vi "medicaoIXV.vi"(0 "Nome da célula":string, 1 "Tipo":string caption="Tipo da célula", 2 "p.d.j":dbl caption="Pontos depois do joelho", 3 "temperatura":dbl caption="Temperatura da célula" format="%#_3g", 4 "nMedições":i16=1 caption="N° medições por ponto" min=1, 5 "Formato":u16(ring) items=[".txt", ".csv"], 6 "nCurvas":i64=1 caption="Nº de curvas" min=1, 7 "p.a.j":dbl caption="Pontos antes do joelho", 8 "Delay(ms)":dbl, 9 "Local":path, 10 "Start":bool, 11 "T.J":dbl caption="Tensão do joelho" step=0.1, 12 "area":dbl caption="Área da célula(cm²)", 13 "Irradiância":dbl caption="Irradiância(W/cm²)", 14 "T.M":dbl caption="Tensão máxima" step=0.1, 15 "print?":bool) -> ()   [LabVIEW 2012]
uses:
  <vilib>/silver_ctls/ArrayMatrixCluster/Real Matrix NI_Silver.ctl
  <vilib>/Utility/file.llb/Write To Spreadsheet File (string).vi
  <vilib>/Utility/file.llb/Write To Spreadsheet File (DBL).vi
  <instrlib>/Agilent 6XXX Series/Agilent 6XXX Series.lvlib
  <vilib>/Analysis/NI_AALBase.lvlib
panel:
  out "Curva atual":dbl
  in  "correcao":bool caption="Correção da curva"
  in  "stopProgram":bool caption="Realizar outra medição"
  out "ON/OFF1":bool caption="ON/OFF"
  out "tensaoFonte":dbl caption="Tensão da fonte (V)"
  out "Temp":dbl caption="Temperatura da célula (°C)" format="%#_3g"
  out "Imp":dbl caption="Imp(A)"
  out "Vmp":dbl caption="Vmp(V)"
  out "Pmp":dbl caption="Pmp(W)"
  out "Icc (A)":dbl
  out "Vca (V)":dbl
  out "IXV":cluster{"Y":dbl[], "Y":dbl[]}[](graph)
  out "vAtual":dbl caption="Tensao Atual (V)"
  out "iAtual":dbl caption="Corrente Atual (A)"
  out "Ponto Atual":i32
  out "tabela 2":T1 caption="TABELA DE DADOS\nTensão(Fonte)      Pontos             Tensao           Corrente"
  in  "stop":bool caption="Parar Medição"
  out "ON/OFF2":bool caption="ON/OFF"
  out "eficiencia":dbl caption="Eficiencia(%)"
  out "FF":dbl
  out "stopLoopMedicoes":bool caption="Parar Medição"
  out "desvio":dbl format="%0.2f"
  out "reset graph":bool=TRUE
  out "tabela":dbl[][](array[numeric])
  in  "CorrenteGraph":dbl
  in  "TensaoGraph":dbl
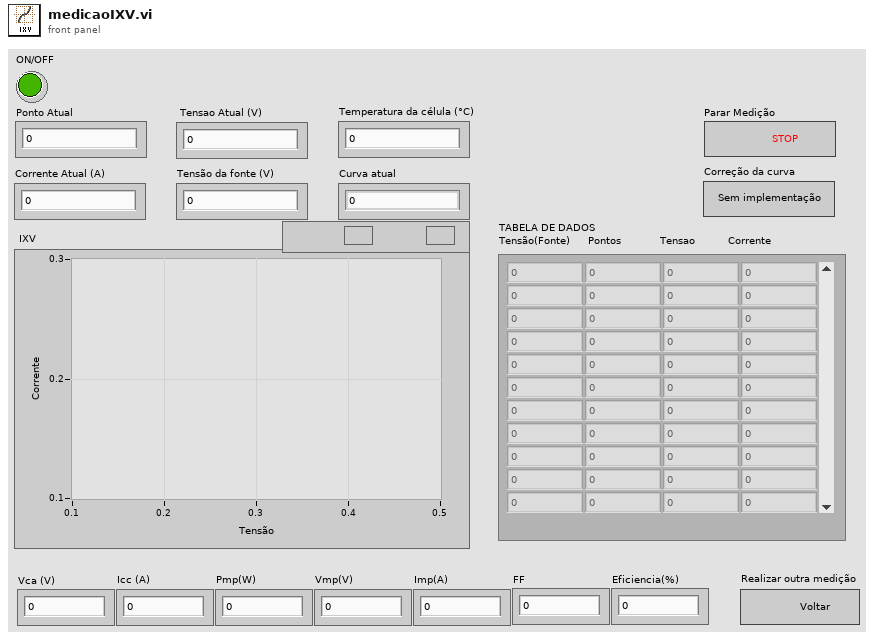
[diagram p1: front panel]
types:
  T1 = typedef "Real Matrix NI_Silver.ctl" = dbl[][]
  T2 = typedef "imagedata.ctl" = cluster{"image type":i32, "image depth":i32, "image":u8[], "mask":u8[], "colors":u32[], "Rectangle":cluster{"left":i16, "top":i16, "right":i16, "bottom":i16}}
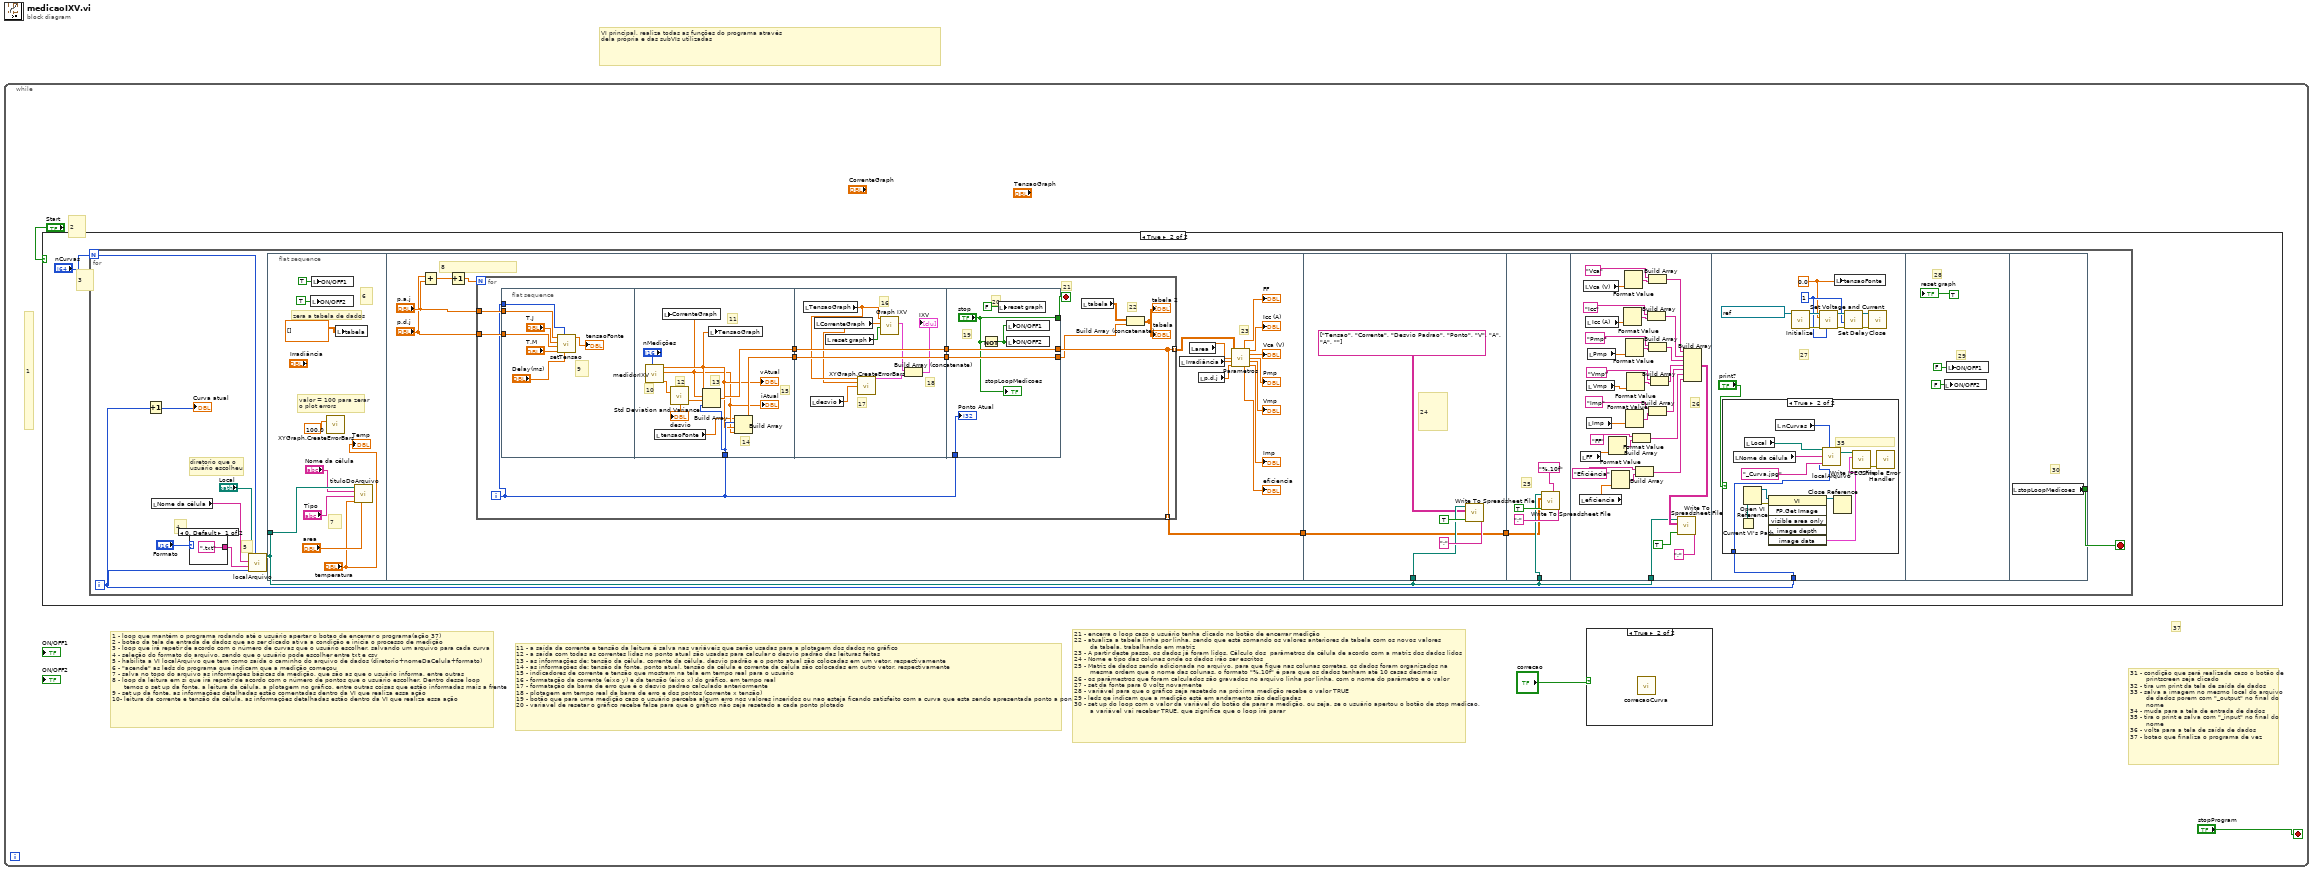
[diagram p0: block diagram]
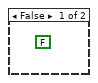
[diagram p3: hidden frame]
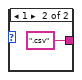
[diagram p4: hidden frame]
diagram:
  # "VI principal, realiza todas as funções do programa através \ndela própria e das subVIs utilizadas"
  n1 = while {
    stop <- "stopProgram" stop-if-true
    # "21 - encerra o loop caso o usuário tenha clicado no botão de encerrar medição\n22 - atualiza a tabela linha por linha, sendo que está somando os valores anteriores da tabela com os novos valores\n        da tabela, trabalhando em matriz\n23 - A partir deste passo, os dados já foram lidos. Cálculo dos  parâmetros da célula de acordo com a matriz dos dados lidos\n24 - Nome e tipo das colunas onde os dados irão ser escritos\n25 - Matriz de dados sendo adicionada no arquivo. para que fique nas colunas corretas, os dados foram organizados na \n        mesma ordem que o nome das colunas. o formato \"%.10f\" é para que os dados tenham até 10 casas decimais\n26 - os parâmestros que foram calculados são gravados no arquivo linha por linha, com o nome do parâmetro e o valor\n27 - set da fonte para 0 volts novamente \n28 - variável para que o gráfico seja resetado na próxima medição recebe o valor TRUE \n29 - leds qe indicam que a medição está em andamento são desligadas\n30 - set up do loop com o valor da variável do botão de parar a medição, ou seja, se o usuário apertou o botão de stop medicao,\n        a variável vai receber TRUE, que significa que o loop irá parar"
    # "11 - a saída da corrente e tensão da leitura é salva nas variáveis que serão usadas para a plotagem dos dados no gráfico\n12 - a saída com todas as correntes lidas no ponto atual são usadas para calcular o desvio padrão das leituras feitas\n13 - as informações de: tensão da célula, corrente da célula, desvio padrão e o ponto atual são colocadas em um vetor, respectivamente\n14 - as informações de: tensão da fonte, ponto atual, tensão da célula e corrente da célula são colocadas em outro vetor, respectivamente\n15 - indicadores de corrente e tensão que mostram na tela em tempo real para o usuário \n16 - formatação da corrente (eixo y) e da tensão (eixo x) do gráfico, em tempo real\n17 - formatação da barra de erro que é o desvio padrao calculado anteriormente\n18 - plotagem em tempo real da barra de erro e dos pontos (corrente x tensão)\n19 - botão que para uma medição caso o usuário perceba algum erro nos valores inseridos ou nao esteja ficando satisfeito com a curva que esta sendo apresentada ponto a ponto\n20 - variavel de resetar o gráfico recebe false para que o gráfico não seja resetado a cada ponto plotado"
    # "1 - loop que mantém o programa rodando até o usuário apertar o botao de encerrar o programa(ação 37)\n2 - botão da tela de entrada de dados que ao ser clicado ativa a condição e inicia o processo de medição\n3 - loop que irá repetir de acordo com o número de curvas que o usuário escolher, salvando um arquivo para cada curva \n4 - seleção do formato do arquivo, sendo que o usuário pode escolher entre txt e csv\n5 - habilita a VI localArquivo que tem como saída o caminho do arquivo de dados (diretorio+nomeDaCelula+formato) \n6 - \"acende\" as leds do programa que indicam que a medição começou\n7 - salva no topo do arquivo as informações básicas da medição, que são as que o usuário informa, entre outras\n8 - loop da leitura em si que irá repetir de acordo com o número de pontos que o usuário escolher. Dentro desse loop\n      temos o set up da fonte, a leitura da célula, a plotagem no gráfico, entre outras coisas que estão informadas mais a frente\n9 - set up da fonte, as informações detalhadas estão comentadas dentro da VI que realiza essa ação\n10- leitura da corrente e tensão da célula. as informações detalhadas estão dentro da VI que realiza essa ação"
    # "31 - condição que será realizada caso o botão de\n        printscreen seja clicado\n32 - tira um print da tela de saída de dados\n33 - salva a imagem no mesmo local do arquivo\n        de dados porem com \"_output\" no final do\n        nome\n34 - muda para a tela de entrada de dados\n35 - tira o print e salva com \"_input\" no final do\n        nome\n36 - volta para a tela de saída de dados \n37 - botao que finaliza o programa de vez"
    # "37"
    # "2"
    # "1"
    n2 = case shown="True" "Start" {
      frame False {
        (unwired) FALSE
      }
      frame True {
        # "3"
        n3 = for {
          N: "nCurvas" -> [w8]
          i -> [w6]
          stop <- w7 stop-if-true
          # "diretorio que o\nusuário escolheu"
          # "5"
          # "4"
          n4 = Increment(x=w6) -> (x+1=→"Curva atual":i32)
          n5 = local read "Nome da célula"() -> (w11:string)
          n6 = case shown="0, Default" "Formato" {
            tunnel: [".txt" ".csv"] -> w10
            frame 0, Default {
            }
            frame 1 {
            }
          }
          n7 = call "localArquivo.vi"("quantidadeDeArquivos"=w8, "nAtualDoArquivo"=w6, "extensão"=w10, "Nome do arquivo"=w11, "Local"="Local") -> ("Path"=w9:path)  [unwired: 6 in]
          n8 = flat-sequence {
            tunnel: w9 -> [w26]
            tunnel: [w38] -> w15
            tunnel: w9 -> [w88]
            tunnel: [w87] -> w14
            tunnel: w15 -> [w87]
            tunnel: w9 -> [w92]
            tunnel: w14 -> [w91]
            tunnel: w9 -> [w104]
            tunnel: w6 -> [w129]
            tunnel: [w154] -> w7
            frame #0 {
              # "zera a tabela de dados"
              # "7"
              # "6"
              # "valor = 100 para zerar\no plot errors"
              n9 = local write "ON/OFF2"(TRUE ("ON/OFF2")) -> ()
              n10 = local write "ON/OFF1"(TRUE ("ON/OFF")) -> ()
              n11 = call "XYGraph.CreateErrorBars.vi"("yTemp"=100.0) -> ()  [unwired: 14 in, 1 out]
              n12 = local write "tabela"(dbl[][] [] ("array")) -> ()
              n13 = call "tituloDoArquivo.vi"("area"="area", "temperatura"="temperatura", "Tipo"="Tipo", "Nome da célula"="Nome da célula", "file path (dialog if empty)"=w26) -> ()  [unwired: 7 in]
              "Temp" <- "temperatura"
            }
            frame #1 {
              # "23"
              # "8"
              n14 = Add(x="p.d.j", y="p.a.j") -> (x+y=w41:dbl)
              n15 = Increment(x=w41) -> (x+1=w42:dbl)
              n16 = for {
                N: w42 -> [_]
                tunnel: [w45] -> w31 mode=indexing
                tunnel: "p.a.j" -> [w47]
                tunnel: "p.d.j" -> [w46]
                tunnel: [w45] -> w38 mode=indexing
                i -> [w43]
                stop <- w50 stop-if-true
                # "22"
                # "21"
                n17 = flat-sequence {
                  tunnel: w43 -> [w61]
                  tunnel: w47 -> [w59]
                  tunnel: w46 -> [w58]
                  tunnel: w43 -> [w67]
                  tunnel: [w69] -> w54
                  tunnel: [w70] -> w53
                  tunnel: [w79] -> w49
                  tunnel: [w78] -> w48
                  tunnel: w53 -> [w78]
                  tunnel: w54 -> [w79]
                  tunnel: [w84] -> w44
                  tunnel: [w85] -> w45
                  tunnel: w49 -> [w85]
                  tunnel: w48 -> [w84]
                  tunnel: w43 -> [w83]
                  tunnel: ["stop"] -> w50
                  frame #0 {
                    # "9"
                    n18 = call "setTensao.vi"("delay(ms)"="Delay(ms)", "Ponto atual"=w61, "T.M"="T.M", "P.D.J"=w58, "T.J"="T.J", "P.A.J"=w59) -> ("output voltage"=→"tensaoFonte":dbl)  [unwired: 5 in]
                  }
                  frame #1 {
                    # "15"
                    # "14"
                    # "13"
                    # "11"
                    # "12"
                    # "10"
                    n19 = call "medidorIXV.vi"("nMedicoes"="nMedições") -> ("Tensao Atual"=w66:dbl, "Corrente Atual"=w65:dbl, "vetorCorrente"=w68:dbl[])  [unwired: 7 in]
                    "iAtual" <- w65
                    "vAtual" <- w66
                    n20 = local read "tensaoFonte"() -> (w62:dbl)
                    n21 = local write "CorrenteGraph"(w65) -> ()
                    n22 = call <vilib>:"Std Deviation and Variance.vi"("X"=w68) -> ("standard deviation"=w64:dbl)  [unwired: 1 in, 2 out]
                    "desvio" <- w64
                    n23 = Build Array(w66, w65, w64, w67) -> (w69:dbl[])
                    n24 = local write "TensaoGraph"(w66) -> ()
                    n25 = Build Array(w62, w67, w66, w65) -> (w70:dbl[])
                  }
                  frame #2 {
                    # "17"
                    # "18"
                    # "16"
                    n26 = local read "TensaoGraph"() -> (w73:dbl)
                    n27 = local read "desvio"() -> (w71:dbl)
                    n28 = local read "CorrenteGraph"() -> (w72:dbl)
                    n29 = local read "reset graph"() -> (w77:bool)
                    n30 = call "XYGraph.CreateErrorBars.vi"("xTemp"=w73, "yTemp"=w72, "errorTemp"=w71) -> ("error bar plot"=w74:cluster{dbl[], dbl[]})  [unwired: 12 in]
                    n31 = call "Graph IXV"("Reset"=w77, "Y Input"=w72, "X Input"=w73) -> ("XY Graph"=w76:cluster{"Y":dbl[], "Y":dbl[]}[])  [unwired: 2 in, 6 out]
                    n32 = Build Array (concatenate)(w76, w74) -> (→"IXV":cluster{"Y":dbl[], "Y":dbl[]}[])
                  }
                  frame #3 {
                    # "20"
                    # "19"
                    n33 = Not(x="stop") -> (.not. x?=w81:bool)
                    n34 = local write "reset graph"(FALSE) -> ()
                    n35 = local write "ON/OFF1"(w81) -> ()
                    n36 = local write "ON/OFF2"(w81) -> ()
                    "Ponto Atual" <- w83
                    "stopLoopMedicoes" <- "stop"
                  }
                }
                n37 = local read "tabela"() -> (w52:dbl[][])
                n38 = Build Array (concatenate)(w52, w44) -> (→"tabela 2" →"tabela":dbl[][])
              }
              n39 = local read "Irradiância"() -> (w29:dbl)
              n40 = local read "area"() -> (w30:dbl)
              n41 = local read "p.d.j"() -> (w32:dbl)
              n42 = call "Parametros.vi"("VetorDeDados"=w31, "area"=w30, "irradiancia"=w29, "pontos"=w32) -> ("FF"=→"FF":dbl, "Icc"=→"Icc (A)":dbl, "Vca"=→"Vca (V)":dbl, "Pmp"=→"Pmp":dbl, "Vmp"=→"Vmp":dbl, "eficiencia"=→"eficiencia":dbl, "Imp"=→"Imp":dbl)  [unwired: 5 in]
            }
            frame #2 {
              # "24"
              n43 = call-poly <vilib>:"Write To Spreadsheet File.vi"("delimiter (\\t)"=";" ("delimiter (\\t)"), "append to file? (new file:F)"=TRUE, "2D data"=string[][] [["Tensao", "Corrente", "Desvio Padrao", "Ponto"], ["V", "A", "A", ""]], "file path (dialog if empty)"=w88) -> ()  [unwired: 4 in, 1 out]
            }
            frame #3 {
              # "25"
              n44 = call-poly <vilib>:"Write To Spreadsheet File.vi"("delimiter (\\t)"=";" ("delimiter (\\t)"), "format (%.3f)"="%.10f", "append to file? (new file:F)"=TRUE, "2D data"=w91, "file path (dialog if empty)"=w92) -> ()  [unwired: 3 in, 1 out]
            }
            frame #4 {
              # "26"
              n45 = local read "eficiencia"() -> (w98:dbl)
              n46 = local read "FF"() -> (w99:dbl)
              n47 = local read "Vca (V)"() -> (w106:dbl)
              n48 = local read "Icc (A)"() -> (w116:dbl)
              n49 = local read "Imp"() -> (w119:dbl)
              n50 = local read "Vmp"() -> (w118:dbl)
              n51 = local read "Pmp"() -> (w117:dbl)
              n52 = Format Value(value (0)=w99) -> (output string=w103:string)  [unwired: 2 in]
              n53 = Format Value(value (0)=w98) -> (output string=w102:string)  [unwired: 2 in]
              n54 = Format Value(value (0)=w116) -> (output string=w109:string)  [unwired: 2 in]
              n55 = Format Value(value (0)=w106) -> (output string=w107:string)  [unwired: 2 in]
              n56 = Format Value(value (0)=w117) -> (output string=w111:string)  [unwired: 2 in]
              n57 = Format Value(value (0)=w119) -> (output string=w115:string)  [unwired: 2 in]
              n58 = Format Value(value (0)=w118) -> (output string=w113:string)  [unwired: 2 in]
              n59 = Build Array("FF" ("string (\"\")"), w103) -> (w101:string[])
              n60 = Build Array("Eficiência" ("string (\"\")"), w102) -> (w100:string[])
              n61 = Build Array("Icc", w109) -> (w121:string[])
              n62 = Build Array("Vca", w107) -> (w120:string[])
              n63 = Build Array("Pmp", w111) -> (w122:string[])
              n64 = Build Array("Imp", w115) -> (w124:string[])
              n65 = Build Array("Vmp", w113) -> (w123:string[])
              n66 = Build Array(w120, w121, w122, w123, w124, w101, w100) -> (w125:string[][])
              n67 = call-poly <vilib>:"Write To Spreadsheet File.vi"("delimiter (\\t)"=";" ("delimiter (\\t)"), "append to file? (new file:F)"=TRUE, "2D data"=w125, "file path (dialog if empty)"=w104) -> ()  [unwired: 4 in, 1 out]
            }
            frame #5 {
              w130 = 0.0 ("voltage (0 V)")
              w133 = u8 1 ("channel (1)")
              # "27"
              n68 = case shown="True" "print?" {
                tunnel: w129 -> [_ w139]
                frame False {
                }
                frame True {
                  # "35"
                  n69 = local read "Nome da célula"() -> (w148:string)
                  n70 = Current VI's Path() -> (path=w142:path)
                  n71 = Open VI Reference(vi path=w142) -> (vi reference=w143:refnum<vi>, error out=w144:errorcluster)  [unwired: 5 in]
                  n72 = local read "Local"() -> (w149:path)
                  n73 = invoke class="VI" method="FP.Get Image"(reference=w143, error in=w144) -> (reference out=w141:refnum<vi>, "image data"=w146:T2)  [unwired: 4 in, 4 out]
                  n74 = local read "nCurvas"() -> (w140:i64)
                  n75 = call "localArquivo.vi"("quantidadeDeArquivos"=w140, "nAtualDoArquivo"=w139, "extensão"="_Curva.jpg", "Nome do arquivo"=w148, "Local"=w149) -> ("Path"=w150:path)  [unwired: 6 in]
                  n76 = Close Reference(reference=w141) -> ()  [unwired: 1 in, 1 out]
                  n77 = call <vilib>:"Write JPEG File.vi"("image data"=w146, "path to JPEG file"=w150) -> ("error out"=w145:errorcluster)  [unwired: 8 in, 1 out]
                  n78 = call <vilib>:"Simple Error Handler.vi"("error in (no error)"=w145) -> ()  [unwired: 4 in, 5 out]
                }
              }
              n79 = call <instrlib>:"Initialize.vi"("VISA resource name"=refnum<visa-resource-name> "GPIB0::5::INSTR") -> ("error out"=w135:errorcluster, "VISA resource name out"=w134:refnum<visa-resource-name>)  [unwired: 9 in]
              n80 = call <instrlib>:"Set Voltage and Current.vi"("channel (1)"=w133, "error in (no error)"=w135, "voltage (0 V)"=w130, "VISA resource name"=w134) -> ("error out"=w136:errorcluster, "VISA resource name out"=w137:refnum<visa-resource-name>)  [unwired: 6 in]
              n81 = local write "tensaoFonte"(w130) -> ()
              n82 = call <instrlib>:"Set Delay.vi"("error in (no error)"=w136, "channel (1)"=w133, "VISA resource name"=w137) -> ("error out"=w131:errorcluster, "VISA resource name out"=w132:refnum<visa-resource-name>)  [unwired: 7 in]
              n83 = call <instrlib>:"Close.vi"("error in (no error)"=w131, "VISA resource name"=w132) -> ()  [unwired: 9 in, 1 out]
            }
            frame #6 {
              # "29"
              # "28"
              n84 = local write "ON/OFF2"(FALSE ("ON/OFF")) -> ()
              n85 = local write "ON/OFF1"(FALSE) -> ()
              "reset graph" <- TRUE
            }
            frame #7 {
              # "30"
              n86 = local read "stopLoopMedicoes"() -> (w154:bool)
            }
          }
        }
      }
    }
    n87 = case shown="True" "correcao" {
      frame False {
      }
      frame True {
        n88 = call "correcaoCurva.vi"() -> ()  [unwired: 12 in]
      }
    }
  }
